vi "echo_client.vi"() -> ()   [LabVIEW 2015]
doc: "Demonstrates how to open a connection to an TCP server, read the data being sent, and display the data on a chart. This VI is designed to stop if the TCP connection is terminated."
panel:
  out "String":string
  out "echo data from server":string
  in  "data to server":string
  in  "Send data":bool
  in  "server-address":string
  in  "Server Closed":string="The server VI closed the connection."
  in  "Stop":bool
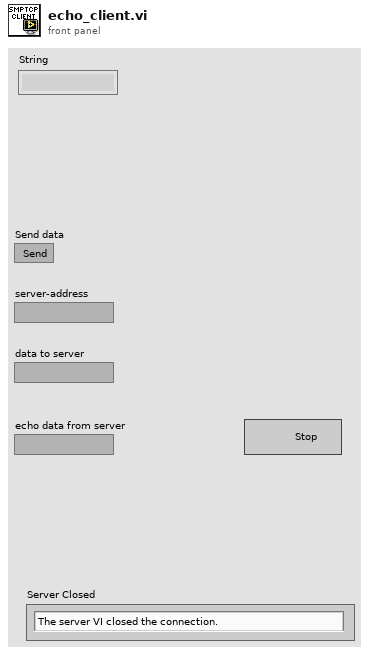
[diagram p1: front panel]
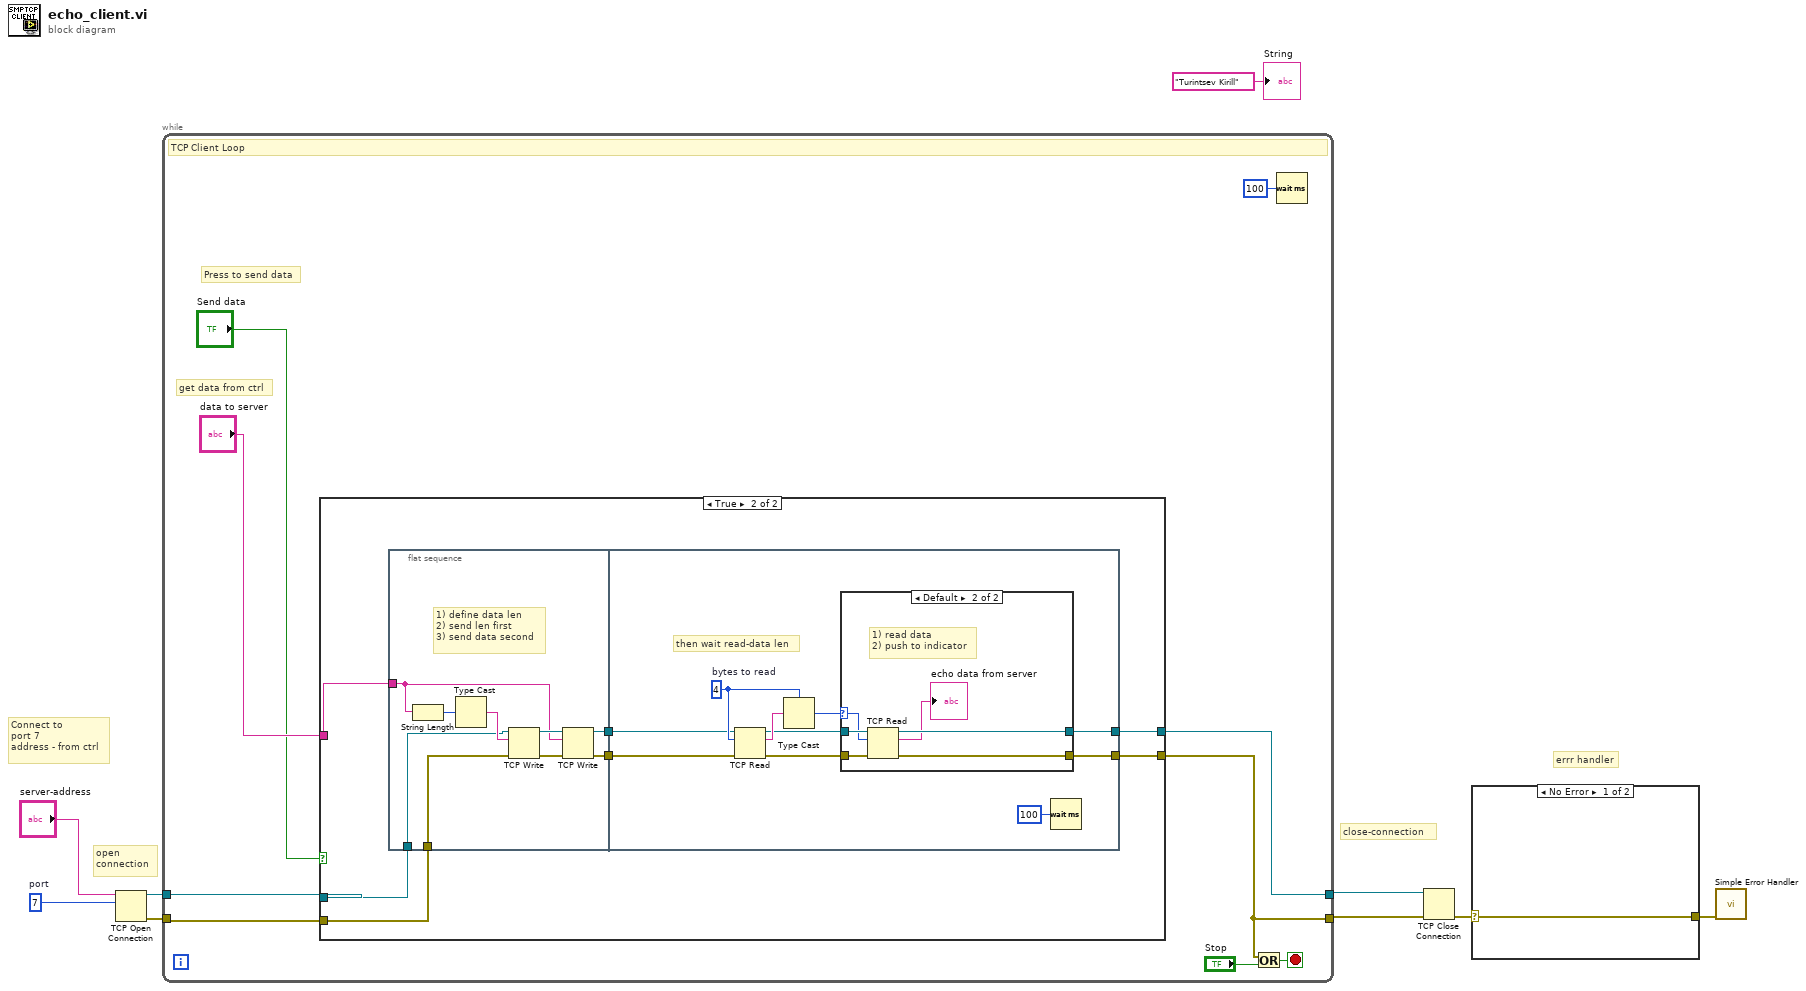
[diagram p0: block diagram]
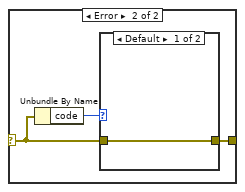
[diagram p2: hidden frame]
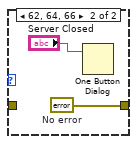
[diagram p3: hidden frame]
diagram:
  w5 = u16 7  # port
  # "errr handler"
  # "close-connection"
  # "open\nconnection"
  # "Connect to\nport 7\naddress - from ctrl"
  n1 = TCP Open Connection(address="server-address", remote port or service name=w5) -> (connection ID=w9:refnum<k5>, error out=w8:errorcluster)  [unwired: 3 in]
  n2 = while {
    tunnel: w8 -> [w13]
    tunnel: w9 -> [w14]
    tunnel: [w12] -> w3
    tunnel: [w11] -> w2
    stop <- w17 stop-if-true
    # "get data from ctrl"
    # "Press to send data"
    # "TCP Client Loop"
    n3 = case shown="True" "Send data" {
      tunnel: "data to server" -> [_ w25]
      tunnel: w14 -> [w20 w22]
      tunnel: w13 -> [w19 w21]
      tunnel: [w20 w27] -> w12
      tunnel: [w19 w26] -> w11
      frame False {
      }
      frame True {
        n4 = flat-sequence {
          tunnel: w25 -> [w32]
          tunnel: [w31] -> w24
          tunnel: [w30] -> w23
          tunnel: w22 -> [w29]
          tunnel: w21 -> [w28]
          tunnel: [w39] -> w27
          tunnel: [w38] -> w26
          tunnel: w23 -> [w40]
          tunnel: w24 -> [w41]
          frame #0 {
            # "1) define data len\n2) send len first\n3) send data second"
            n5 = String Length(string=w32) -> (length=w34:i32)
            n6 = Type Cast(x=w34) -> (*(type *) &x=w33:string)  [unwired: 1 out]
            n7 = TCP Write(connection ID=w29, data in=w33, error in (no error)=w28) -> (connection ID out=w36:refnum<k5>, error out=w35:errorcluster)  [unwired: 2 out]
            n8 = TCP Write(connection ID=w36, data in=w32, error in (no error)=w35) -> (connection ID out=w31:refnum<k5>, error out=w30:errorcluster)  [unwired: 2 out]
          }
          frame #1 {
            w43 = 4  # bytes to read
            # "then wait read-data len"
            n9 = TCP Read(connection ID=w41, bytes to read=w43, error in (no error)=w40) -> (connection ID out=w45:refnum<k5>, data out=w46:string, error out=w44:errorcluster)  [unwired: 2 in]
            n10 = Type Cast(type=w43, x=w46) -> (*(type *) &x=w42:i32)
            n11 = case shown="Default" w42 {
              selector: w42 -> [_ w50]
              tunnel: w45 -> [w48 w54]
              tunnel: w44 -> [w47 w53]
              tunnel: [w48 w52] -> w39
              tunnel: [w47 w51] -> w38
              frame ..0 {
                # "The server has not written any data"
              }
              frame Default {
                # "1) read data\n2) push to indicator"
                n12 = TCP Read(connection ID=w54, bytes to read=w50, error in (no error)=w53) -> (connection ID out=w52:refnum<k5>, data out=→"echo data from server":string, error out=w51:errorcluster)  [unwired: 2 in]
              }
            }
            n13 = Wait (ms)(milliseconds to wait=u32 100) -> ()  [unwired: 1 out]
          }
        }
      }
    }
    n14 = Or(x=w11, y="Stop") -> (x .or. y?=w17:bool)
    n15 = Wait (ms)(milliseconds to wait=u32 100) -> ()  [unwired: 1 out]
  }
  n16 = TCP Close Connection(connection ID=w3, error in (no error)=w2) -> (error out=w7:errorcluster)  [unwired: 1 in, 1 out]
  n17 = case shown="No Error" w7 {
    selector: w7 -> [w55 w57]
    tunnel: [w55 w56] -> w6
    frame No Error {
    }
    frame Error {
      n18 = Unbundle By Name(w57) -> ("code"=w58:i32)
      n19 = case shown="Default" w58 {
        tunnel: w57 -> [w59 _]
        tunnel: [w59 w61] -> w56
        frame Default {
        }
        frame 62, 64, 66 {
          w61 = errorcluster {"status"=FALSE, "code"=0, "source"=""}  # No error
          n20 = One Button Dialog(message="Server Closed") -> ()  [unwired: 1 in, 1 out]
        }
      }
    }
  }
  n21 = call <vilib>:"Simple Error Handler.vi"("error in (no error)"=w6) -> ()  [unwired: 4 in, 5 out]
  "String" <- "Turintsev Kirill" ("String")
